vi "Add Measurement Plugin Controls.vi"(11 "error in (no error)":errorcluster) -> (15 "error out":errorcluster)   [LabVIEW 2021, in "Migrator.lvlib"]
uses:
  Migrator.lvlib
  Migrator Reusables/Migrator Reusables.lvlib
  Path Functions/Path Functions.lvlib
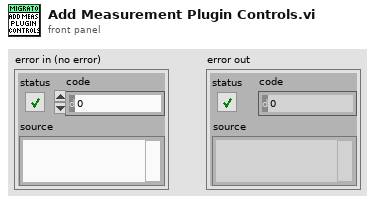
[diagram p1: front panel]
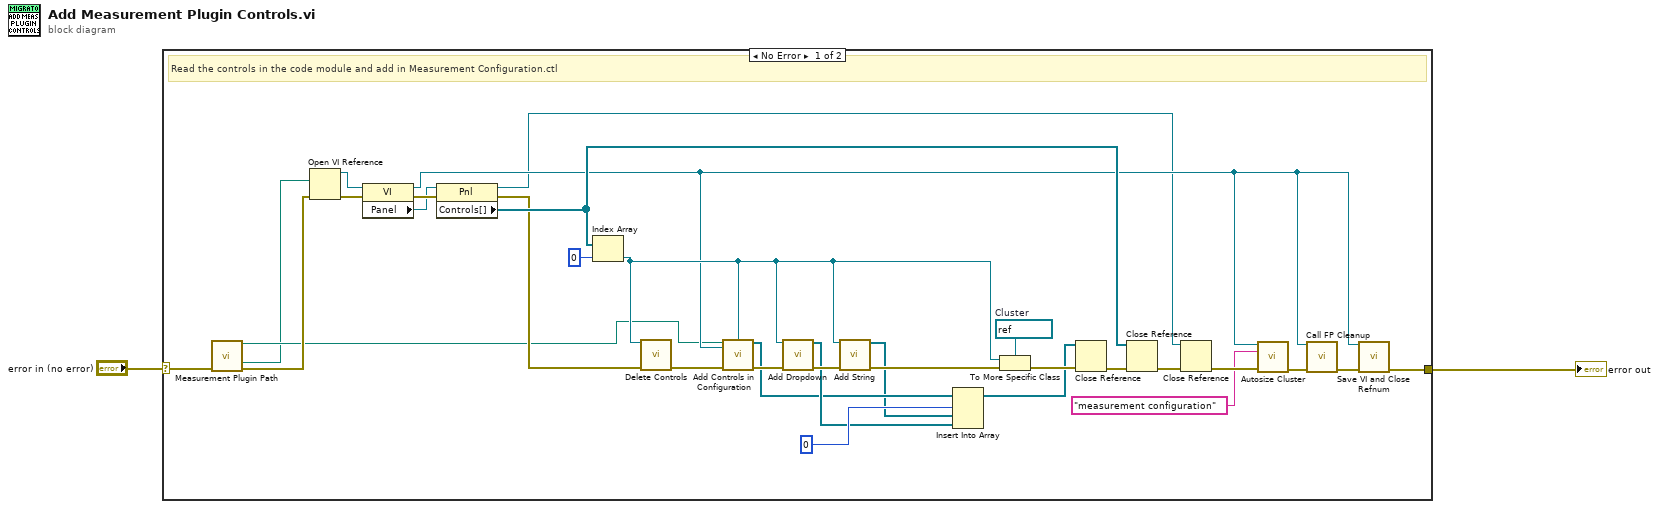
[diagram p0: block diagram]
diagram:
  n1 = case shown="No Error" "error in (no error)" {
    selector: "error in (no error)" -> [w6 w35]
    tunnel: [w29 w35] -> w1
    frame No Error {
      w28 = refnum<vi> refnum  # Cluster
      # "Read the controls in the code module and add in Measurement Configuration.ctl"
      n2 = call "Measurement Plugin Path.vi"("error in (no error)"=w6) -> ("New Code Module"=w4:path, "Input Controls"=w3:path, "error out"=w5:errorcluster)  [unwired: 2 in, 10 out]
      n3 = Open VI Reference(vi path=w3, error in (no error)=w5) -> (vi reference=w10:refnum<vi>, error out=w30:errorcluster)  [unwired: 4 in]
      n4 = property class="VI"(reference=w10, error in=w30) -> (reference out=w9:refnum<vi>, error out=w34:errorcluster, "Panel"=w8:refnum<vi>)
      n5 = property class="Pnl"(reference=w8, error in=w34) -> (reference out=w7:refnum<vi>, error out=w18:errorcluster, "Controls[]"=w23:refnum<vi>[])
      n6 = Index Array(array=w23, index=0) -> (element=w17:refnum<vi>)
      n7 = call "Delete Controls.vi"("Control in"=w17, "error in (no error)"=w18) -> ("error out"=w19:errorcluster)  [unwired: 13 in]
      n8 = call "Add Controls in Configuration.vi"("New Code Module"=w4, "vi reference"=w9, "Configuration Ctl Refnum"=w17, "error in (no error)"=w19) -> ("Controls Reference"=w13:refnum<vi>[], "error out"=w20:errorcluster)  [unwired: 10 in]
      n9 = call "Add Dropdown.vi"("Control in"=w17, "error in (no error)"=w20) -> ("ComboBox out"=w14:refnum<vi>[], "error out"=w15:errorcluster)  [unwired: 12 in]
      n10 = call "Add String.vi"("Control in"=w17, "error in (no error)"=w15) -> ("ComboBox out"=w11:refnum<vi>[], "error out"=w16:errorcluster)  [unwired: 12 in]
      n11 = Insert Into Array(array=w13, index=0, new element #1=w11, new element #2=w14) -> (w12:refnum<vi>[])
      n12 = To More Specific Class(target class=w28, reference=w17, error in=w16) -> (error out=w26:errorcluster)  [unwired: 1 out]
      n13 = Close Reference(reference=w12, error in (no error)=w26) -> (error out=w22:errorcluster)
      n14 = Close Reference(reference=w23, error in (no error)=w22) -> (error out=w21:errorcluster)
      n15 = Close Reference(reference=w7, error in (no error)=w21) -> (error out=w32:errorcluster)
      n16 = call "Autosize Cluster.vi"("VI Refnum"=w9, "name"="measurement configuration" ("name/order"), "error in (no error)"=w32) -> ("error out"=w24:errorcluster)  [unwired: 12 in]
      n17 = call "Call FP Cleanup.vi"("VI"=w9, "error in (no error)"=w24) -> ("error out"=w25:errorcluster)  [unwired: 13 in]
      n18 = call "Save VI and Close Refnum.vi"("VI Refnum"=w9, "error in"=w25) -> ("error out"=w29:errorcluster)  [unwired: 13 in]
    }
    frame Error {
    }
  }
  "error out" <- w1
